vi "CMI ckd2 Open.vi"(8 "error in":errorcluster, 11 "session":T1) -> (0 "error out":errorcluster, 2 "read buffer":string, 3 "session out":T1)   [LabVIEW 2020, in "AWG.lvlib"]
doc: "Initializes CMI clock divider v2."
uses:
  AWG.lvlib
  CMI ckd2 Session.ctl
  CMI ckd2 Source Mode.ctl
  <vilib>/Utility/error.llb/Error Cluster From Error Code.vi
  <vilib>/ErrorRing/Error Ring.xnode
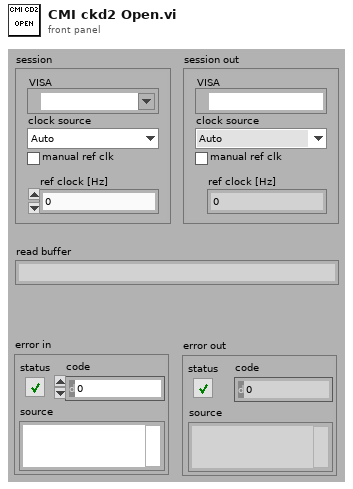
[diagram p1: front panel]
types:
  T1 = typedef "AWG.lvlib/CMI ckd2 Session.ctl" = cluster{"VISA":refnum<visa-resource-name>, "clock source":T2, "manual ref clk":bool, "ref clock [Hz]":dbl}
  T2 = typedef "AWG.lvlib/CMI ckd2 Source Mode.ctl" = enum16{"Auto", "LF clock", "HF clock", "Internal"}
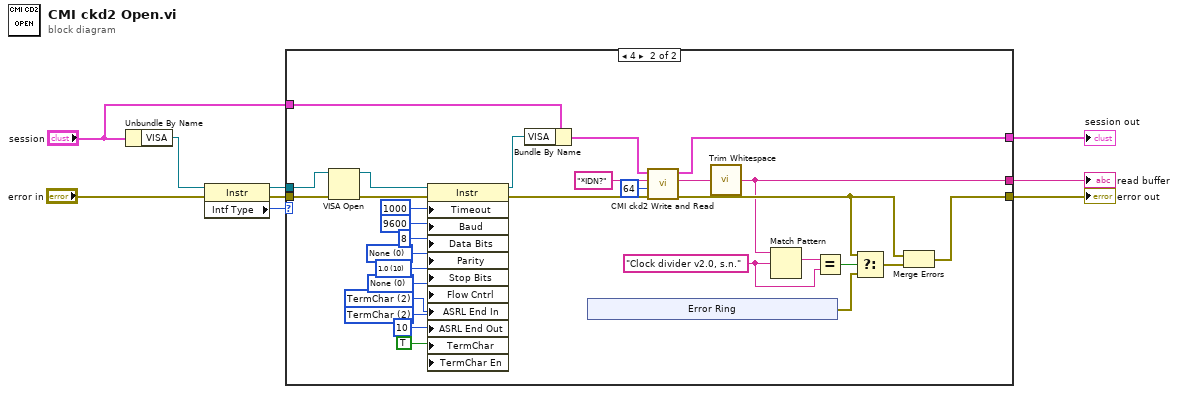
[diagram p0: block diagram]
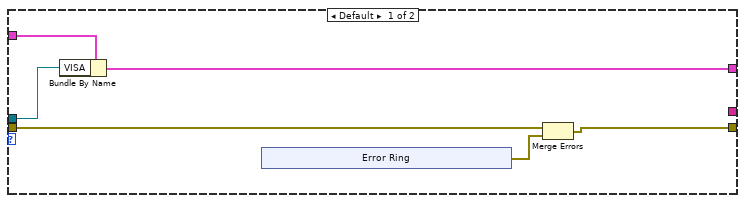
[diagram p2: hidden frame]
diagram:
  n1 = Unbundle By Name("session") -> ("VISA"=w6:refnum<visa-resource-name>)
  n2 = property class="Instr"(reference=w6, error in="error in") -> (reference out=w4:refnum<visa-resource-name>, error out=w5:errorcluster, "Intf Type"=w3:u16)
  n3 = case shown="4" w3 {
    tunnel: w5 -> [w15 w28]
    tunnel: w4 -> [w12 w27]
    tunnel: [w10 w38] -> w1
    tunnel: [w13 w31] -> w9
    tunnel: [_ w29] -> w8
    tunnel: "session" -> [w11 w23]
    frame Default {
      n4 = Bundle By Name(cluster=w11, "VISA"=w12) -> (w10:T1)
      n5 = xnode "Error Ring"() -> ("error out"=w14:errorcluster)
      n6 = Merge Errors(w15, w14) -> (w13:errorcluster)
    }
    frame 4 {
      w36 = "Clock divider v2.0, s.n." ("regular expression")
      w44 = u16 2 items=["None", "Last Bit", "TermChar", "Break"] ("Serial Settings:End Mode for Writes")
      w45 = u16 2 items=["None", "Last Bit", "TermChar"] ("Serial Settings:End Mode for Reads")
      w46 = u16 0 items=["None", "XON/XOFF", "RTS/CTS", "XON/XOFF & RTS/CTS", "DTR/DSR", "XON/XOFF & DTR/DSR"] ("Serial Settings:Flow Control")
      w47 = u16 10 items=["1.0"=10, "1.5"=15, "2.0"=20] ("Serial Settings:Stop Bits")
      w48 = u16 0 items=["None", "Odd", "Even", "Mark", "Space"] ("Serial Settings:Parity")
      n7 = VISA Open(error in (no error)=w28, VISA resource name=w27) -> (VISA resource name=w25:refnum<visa-resource-name>, error out=w26:errorcluster)  [unwired: 3 in]
      n8 = property class="Instr"(reference=w25, error in=w26, "Timeout"=u32 1000 ("General Settings:Timeout Value"), "Baud"=u32 9600 ("Serial Settings:Baud Rate"), "Data Bits"=u16 8 ("Serial Settings:Data Bits"), "Parity"=w48, "Stop Bits"=w47, "Flow Cntrl"=w46, "ASRL End In"=w45, "ASRL End Out"=w44, "TermChar"=u8 10 ("Message Based Settings:Termination Character"), "TermChar En"=TRUE ("Message Based Settings:Termination Character Enable")) -> (reference out=w24:refnum<visa-resource-name>, error out=w40:errorcluster)
      n9 = Bundle By Name(cluster=w23, "VISA"=w24) -> (w21:T1)
      n10 = xnode "Error Ring"() -> ("error out"=w34:errorcluster)
      n11 = call "CMI ckd2 Write and Read.vi"("error in"=w40, "read byte count (0 - no receive)"=u32 64, "command"="*IDN?" ("write buffer"), "session"=w21) -> ("error out"=w32:errorcluster, "read buffer"=w30:string, "session out"=w38:T1)  [unwired: 5 in]
      n12 = call <vilib>:"Trim Whitespace.vi"("string"=w30) -> ("trimmed string"=w29:string)  [unwired: 1 in]
      n13 = Match Pattern(string=w29, regular expression=w36) -> (match substring=w37:string)  [unwired: 1 in, 3 out]
      n14 = Equal?(x=w37, y=w36) -> (x = y?=w35:bool)
      n15 = Select(t=w32, s=w35, f=w34) -> (s? t:f=w33:errorcluster)
      n16 = Merge Errors(w32, w33) -> (w31:errorcluster)
    }
  }
  "error out" <- w9
  "read buffer" <- w8
  "session out" <- w1
